vi "FPGA.vi"() -> ()   [LabVIEW 2020]
uses:
  <vilib>/Platform/TimedLoop/XDataNode/timing_clust.ctl
  <vilib>/Platform/TimedLoop/XDataNode/nitl_modes.ctl
  <vilib>/Platform/TimedLoop/XDataNode/wakeup.ctl
  <vilib>/rvi/Analysis/measure/FFT/simModelSupport/niFPGA FFT Sim Properties.ctl
  <vilib>/rvi/Analysis/measure/FFT/simModelSupport/niFPGA FFT Sim Types.ctl
  <vilib>/rvi/Analysis/measure/FFT/simModelSupport/niFpgaFFTSimArithmeticProperties.ctl
  <vilib>/rvi/Analysis/measure/FFT/simModelSupport/niFpgaFFTSimDfxp.ctl
  <vilib>/fxp/LVFixedPointQuantizationPolicyTypeDef.ctl
  <vilib>/rvi/DataTransferAndStorage/Container/Common/niFpgaContainerGetUniqueNameForEmu.vi
  <vilib>/rvi/DataTransferAndStorage/Container/Common/niFpgaContainerSetEmuInfo.vi
  <vilib>/rvi/eio/common/nirviEmuReportErrorAndStop.vi
  <vilib>/rvi/eio/common/nirviEmuTemplateMethod_errors.vi
  <vilib>/rvi/DataTransferAndStorage/Container/Common/niFpgaContainerExecOnDevCompGetState.vi
  <vilib>/rvi/Emulation/niFpgaEmulationIsFPGAContextNoSignature.vi
  <vilib>/rvi/Emulation/niFpgaSctlEmulationGetInTimedLoop.vi
  <vilib>/rvi/errors/niFpgaSetErrorForExecOnDevCompSimple.vi
  <vilib>/rvi/FIFO/Fifo_Resource/nirvififoEmulationSetSize.vi
  <vilib>/rvi/FIFO/Fifo_Resource/nirviFifoEmulationQueueMgr.vi
  <instcachedir>/0/nirviFifoEmulationQueueMgr_E5CAEC123FF24DC58D834DCA3CDAA9B5.lvgen/nirviFifoEmulationQueueMgr_E5CAEC123FF24DC58D834DCA3CDAA9B5_003.vi
  <vilib>/rvi/FIFO/Fifo_Resource/nirvififoEmulationDetermineInputValidOut.vi
  <vilib>/rvi/FIFO/Fifo_Resource/nirvififoEmulationCreateLock.vi
  <vilib>/rvi/Emulation/niFpgaProcessEmulError.vi
  <vilib>/rvi/FIFO/Fifo_Resource/nirvififoEmulationObtainLock.vi
  <vilib>/rvi/FIFO/Fifo_Resource/nirvififoEmulationReleaseLock.vi
  <vilib>/rvi/occurrence/nirviWaitOnOccurrenceBase.vi
  <vilib>/rvi/errors/nirviReportUnexpectedCaseInternalError.vi
  <vilib>/rvi/errors/nirviReportUnexpectedCaseInternalError (U32).vi
  <vilib>/Utility/error.llb/Clear Errors.vi
  <vilib>/rvi/interface/RandomDataEmulation/niFpgaRandomDataHandleErrors.vi
  <vilib>/rvi/Emulation/niFpgaEmulationReportErrorSimple.vi
  <vilib>/rvi/Emulation/niFpgaGetClockAttributes.vi
  <vilib>/rvi/Emulation/niFpgaCriticalErrorInLSC.vi
  <vilib>/rvi/Analysis/measure/FFT/simModelSupport/niFpgaFFTSimModelCore.vi
  <vilib>/rvi/LocalResourceManager/LocalResourceManager.xnode
  <vilib>/eio/EIONode/EIONode.xnode
  <vilib>/rvi/DataTransferAndStorage/Container/XNode/niFpgaContainer.xnode
  <vilib>/rvi/FIFO/Fifo_Resource/niFpgaFifoEmulationRefIn.vi
  <vilib>/Platform/TimedLoop/XDataNode/XDataNode.xnode
  <vilib>/rvi/interface/RandomDataEmulation/nirviRandomDataFpgaReadWriteTemplate.vi
  <vilib>/rvi/Analysis/measure/FFT/XNode/niFpgaFFT.xnode
  <vilib>/rvi/FXPMathLib/FxpInterpret/XNode/nifxpmath_Interpret.xnode
  <vilib>/Platform/TimedLoop/XDataNode/XDNodeRunTimeDep.lvlib
panel:
  out "Timed Out? FIFO out index 2":bool
  out "Timed Out? FIFO out IMG 2":bool
  out "Timed Out? FIFO out REAL 2":bool
  in  "FFT loop iterations":i32
  in  "auto stop":bool
  out "FFT time (uSec)":u32
  out "data collection time (uSec)":u32
  in  "Loop number":i32
  out "Element":fxp<+/-,24,7>
  in  "Rate (uSec)":u32 caption="Count(uSec)"
  out "Timed Out?":bool
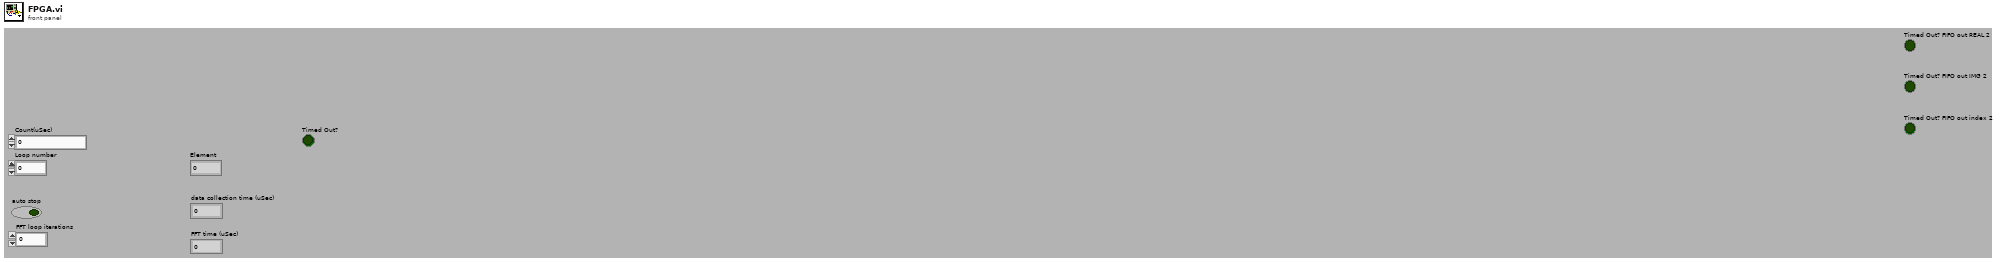
[diagram p1: front panel]
types:
  T1 = typedef "XDNodeRunTimeDep.lvlib/timing_clust.ctl" = cluster{"Expected End [f-1]":u64, "Actual End [f-1]":u64, "Finished Late? [f-1]":bool, "Expected End [i-1]":u64, "Actual End [i-1]":u64, "Finished Late? [i-1]":bool, "Expected Start [i]":u64, "Actual Start [i]":u64, "Expected Start [f]":u64, "Actual Start [f]":u64, "Source Name":string, "Structure Name":string, "Period":i64, "Deadline":i64, "Offset":i64, "Start":i64, "Priority":i32, "Timeout":i32, "Mode":T2, "Wakeup Reason":T3, "Error":errorcluster, "Source Type":string, "Secondary Source Type":string, "Global End Time":u64, "Global Start Time":u64, "Frame Duration":u64, "Iteration Duration":u64, "Assigned CPU":i32, "I/O Scan Engine Mode":u32}
  T2 = typedef "XDNodeRunTimeDep.lvlib/nitl_modes.ctl" = enum32{"No Change", "Process missed periods, maintain original phase", "Discard missed periods, maintain original phase", "Process missed periods, ignore original phase", "Discard missed periods, ignore original phase"}
  T3 = typedef "XDNodeRunTimeDep.lvlib/wakeup.ctl" = enum32{"Normal", "Aborted", "Asynchronous wakeup", "Timing source error", "Timed loop error", "Timeout"}
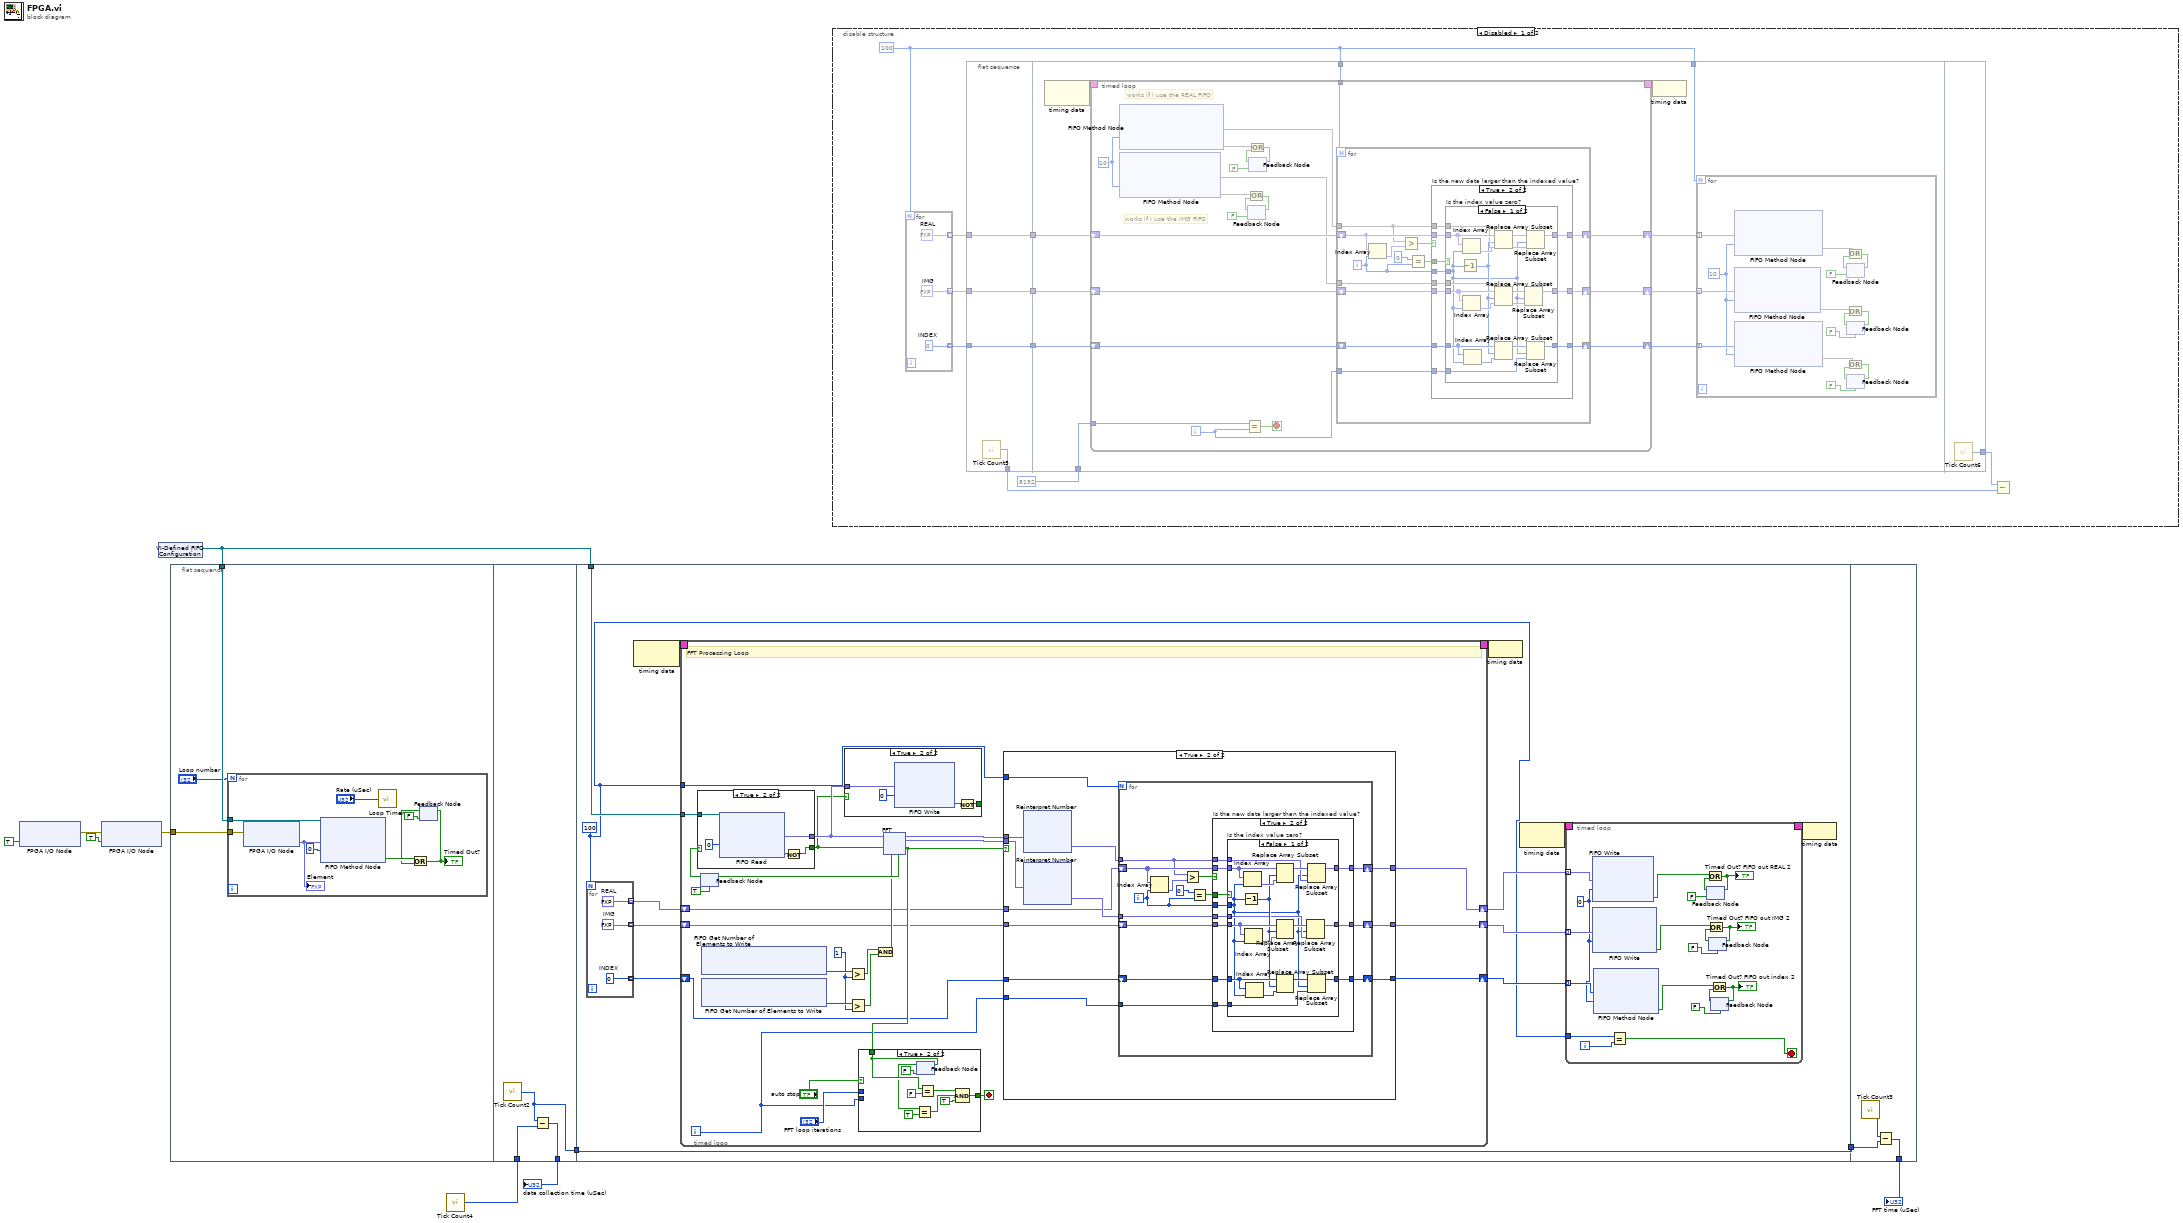
[diagram p0: block diagram]
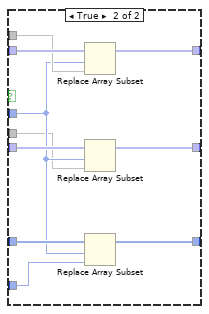
[diagram p3: hidden frame]
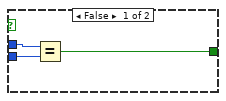
[diagram p5: hidden frame]
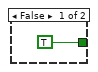
[diagram p6: hidden frame]
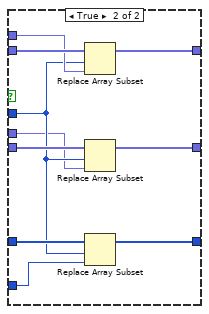
[diagram p9: hidden frame]
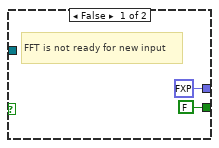
[diagram p10: hidden frame]
diagram:
  n1 = xnode "FPGA I/O Node"("Mod1/Stop"=TRUE) -> ("error out"=w3:errorcluster)  [unwired: 2 in, 1 out]
  n2 = xnode "FPGA I/O Node"("error in"=w3, "Mod1/Start"=TRUE) -> ("error out"=w2:errorcluster)  [unwired: 1 in, 1 out]
  n3 = xnode "VI-Defined FIFO Configuration"() -> ("FIFO Out"=w10:refnum<k21>)
  n4 = flat-sequence {
    tunnel: w10 -> [w13]
    tunnel: w2 -> [w11]
    tunnel: [w25] -> w9
    tunnel: [w24] -> w8
    tunnel: w1 -> [w23]
    tunnel: w10 -> [w36]
    tunnel: w8 -> [w35]
    tunnel: [w35] -> w7
    tunnel: w7 -> [w216]
    tunnel: [w215] -> w6
    frame #0 {
      n5 = for {
        N: "Loop number" -> [_]
        tunnel: w13 -> [w22]
        tunnel: w11 -> [w21]
        n6 = xnode "FPGA I/O Node"("error in"=w21) -> ("Mod1/AI0"=w15:fxp<+/-,24,7>)  [unwired: 1 in, 2 out]
        "Element" <- w15
        n7 = xnode ("FIFO Method Node")("Element"=w15, "Timeout"=0, "FIFO In"=w22) -> ("Timed Out?"=w19:bool)  [unwired: 1 in, 2 out]
        n8 = call "Loop Timer"("Count(uSec)"="Rate (uSec)") -> ()  [unwired: 1 out]
        n9 = feedback #1(FALSE) -> (w18:bool)
        n10 = Or(x=w19, y=w18) -> (x .or. y?=w17:bool)
        "Timed Out?" <- w17
        n11 = feedback-in #1(w17) -> ()
      }
    }
    frame #1 {
      n12 = call "Tick Count2"() -> ("Tick Count(uSec)"=w24:u32)
      n13 = Subtract(x=w24, y=w23) -> (x-y=w25:u32)
    }
    frame #2 {
      w26 = 100
      n14 = for {
        N: w26 -> [_]
        tunnel: [w64] -> w34 mode=indexing
        tunnel: [w63] -> w29 mode=indexing
        tunnel: [w62] -> w33 mode=indexing
        w62 = fxp<+/-,32,21> 0.0  # IMG
        w63 = 0  # INDEX
        w64 = fxp<+/-,32,21> 0.0  # REAL
      }
      n15 = node-c288() -> (w38:T1)  [unwired: 1 in]
      n16 = timed-loop {
        timing: w38 -> [_]
        timing-out: [_] -> w37
        tunnel: w36 -> [w87]
        tunnel: w26 -> [w66]
        shift-right: [w67] -> w30
        shift-left: w29 -> [w65]
        shift-right: [w68] -> w32
        shift-left: w33 -> [w71]
        shift-right: [w69] -> w31
        shift-left: w34 -> [w72]
        i -> [w70]
        stop <- w77 stop-if-true
        w82 = u32 1 ("y")
        # "FFT Processing Loop"
        n17 = feedback #2(TRUE ("ready for input")) -> (w90:bool)
        n18 = case shown="True" w90 {
          tunnel: [FALSE w209] -> w79
          tunnel: [fxp<+/-,16,5> 0.0 ("Element") w210] -> w89
          tunnel: w87 -> [_ w206]
          frame False {
            # "FFT is not ready for new input"
          }
          frame True {
            n19 = xnode ("FIFO Read")("Timeout"=0, "FIFO In"=w206) -> ("Element"=w210:fxp<+/-,24,7>, "Timed Out?"=w208:bool)  [unwired: 1 out]
            n20 = Not(x=w208) -> (.not. x?=w209:bool)
          }
        }
        n21 = xnode ("FIFO Get Number of Elements to Write")() -> ("Number of Elements to Write"=w84:u32)  [unwired: 1 in, 1 out]
        n22 = xnode ("FIFO Get Number of Elements to Write")() -> ("Number of Elements to Write"=w83:u32)  [unwired: 1 in, 1 out]
        n23 = case shown="True" w79 {
          tunnel: w89 -> [_ w104]
          tunnel: [TRUE ("Timed Out?") w105] -> _
          frame False {
          }
          frame True {
            n24 = xnode ("FIFO Write")("Element"=w104, "Timeout"=0) -> ("Timed Out?"=w106:bool)  [unwired: 1 in, 1 out]
            n25 = Not(x=w106) -> (.not. x?=w105:bool)
          }
        }
        n26 = Greater?(x=w84, y=w82) -> (0:w81:bool)
        n27 = Greater?(x=w83, y=w82) -> (0:w80:bool)
        n28 = Compound Arithmetic op=AND(w81, w80) -> (w78:bool)
        n29 = xnode "FFT"("real data in"=w89, "input valid"=w79, "ready for output"=w78) -> ("ready for input"=w88:bool, "real data out"=w86:fxp<+/-,32,21>, "imaginary data out"=w76:fxp<+/-,32,21>, "output valid"=w73:bool)  [unwired: 2 in, 1 out]
        n30 = feedback-in #2(w88) -> ()
        n31 = case shown="True" "auto stop" {
          tunnel: w73 -> [_ w101]
          tunnel: [w91 w94] -> w77
          tunnel: w70 -> [w93 _]
          tunnel: "FFT loop iterations" -> [w92 _]
          frame False {
            n32 = Equal?(x=w92, y=w93) -> (x = y?=w91:bool)
          }
          frame True {
            n33 = feedback #3(FALSE) -> (w98:bool)
            n34 = Equal?(x=w98, y=TRUE) -> (x = y?=w96:bool)
            n35 = feedback-in #3(w101) -> ()
            n36 = Equal?(x=w101, y=FALSE) -> (x = y?=w97:bool)
            n37 = Compound Arithmetic op=AND(w97, w96, TRUE ("value")) -> (w94:bool)
          }
        }
        n38 = case shown="True" w73 {
          tunnel: w86 -> [_ w148]
          tunnel: w76 -> [_ w147]
          tunnel: w72 -> [w136 w144]
          tunnel: w71 -> [w135 w143]
          tunnel: w65 -> [w134 w142]
          tunnel: w70 -> [_ w141]
          tunnel: [w136 w140] -> w69
          tunnel: [w135 w139] -> w68
          tunnel: [w134 w138] -> w67
          tunnel: w66 -> [_ w137]
          frame False {
          }
          frame True {
            n39 = xnode "Reinterpret Number"("x"=w148) -> ("y"=w146:fxp<+/-,32,21>)
            n40 = xnode "Reinterpret Number"("x"=w147) -> ("y"=w145:fxp<+/-,32,21>)
            n41 = for {
              N: w137 -> [_]
              tunnel: w146 -> [w159]
              shift-right: [w158] -> w140
              shift-left: w144 -> [w160]
              tunnel: w141 -> [w156]
              shift-right: [w154] -> w138
              shift-left: w142 -> [w155]
              shift-right: [w151] -> w139
              shift-left: w143 -> [w150]
              tunnel: w145 -> [w149]
              i -> [w157]
              n42 = Index Array(array=w160, index=w157) -> (element=w162:fxp<+/-,32,21>)
              n43 = Greater?(x=w159, y=w162) -> (0:w161:bool)
              n44 = Equal?(x=0, y=w157) -> (x = y?=w152:bool)
              n45 = case "Is the new data larger than the indexed value?" shown="True" w161 {
                tunnel: w160 -> [w165 w175]
                tunnel: w152 -> [_ w176]
                tunnel: w159 -> [_ w174]
                tunnel: w157 -> [_ w173]
                tunnel: [w165 w172] -> w158
                tunnel: w156 -> [_ w171]
                tunnel: w155 -> [w164 w170]
                tunnel: [w164 w169] -> w154
                tunnel: [w163 w168] -> w151
                tunnel: w150 -> [w163 w167]
                tunnel: w149 -> [_ w166]
                frame False {
                }
                frame True {
                  n46 = case "Is the index value zero?" shown="False" w176 {
                    tunnel: w175 -> [w193 w203]
                    tunnel: w174 -> [w190 w202]
                    tunnel: w173 -> [w177 w196]
                    tunnel: [w189 w201] -> w172
                    tunnel: w171 -> [w184 w200]
                    tunnel: w170 -> [w186 w199]
                    tunnel: [w185 w198] -> w169
                    tunnel: [w179 w194] -> w168
                    tunnel: w167 -> [w183 w197]
                    tunnel: w166 -> [w178 w195]
                    frame False {
                      n47 = Decrement(x=w177) -> (x-1=w181:i32)
                      n48 = Index Array(array=w193, index=w177) -> (element=w192:fxp<+/-,32,21>)
                      n49 = Index Array(array=w183, index=w177) -> (element=w182:fxp<+/-,32,21>)
                      n50 = Index Array(array=w186, index=w177) -> (element=w188:i32)
                      n51 = Replace Array Subset(array=w193, new element=w192, index=w181) -> (w191:fxp<+/-,32,21>[])
                      n52 = Replace Array Subset(array=w183, new element=w182, index=w181) -> (w180:fxp<+/-,32,21>[])
                      n53 = Replace Array Subset(array=w186, new element=w188, index=w181) -> (w187:i32[])
                      n54 = Replace Array Subset(array=w180, new element=w178, index=w177) -> (w179:fxp<+/-,32,21>[])
                      n55 = Replace Array Subset(array=w191, new element=w190, index=w177) -> (w189:fxp<+/-,32,21>[])
                      n56 = Replace Array Subset(array=w187, new element=w184, index=w177) -> (w185:i32[])
                    }
                    frame True {
                      n57 = Replace Array Subset(array=w203, new element=w202, index=w196) -> (w201:fxp<+/-,32,21>[])
                      n58 = Replace Array Subset(array=w197, new element=w195, index=w196) -> (w194:fxp<+/-,32,21>[])
                      n59 = Replace Array Subset(array=w199, new element=w200, index=w196) -> (w198:i32[])
                    }
                  }
                }
              }
            }
          }
        }
      }
      n60 = node-c288(w37) -> ()
      n61 = node-c288() -> (w28:T1)  [unwired: 1 in]
      n62 = timed-loop {
        tunnel: w32 -> [w57] mode=indexing
        tunnel: w31 -> [w56] mode=indexing
        tunnel: w30 -> [w46] mode=indexing
        timing: w28 -> [_]
        timing-out: [_] -> w27
        tunnel: w26 -> [w40]
        i -> [w41]
        stop <- w39 stop-if-true
        w45 = 0 ("Timeout")
        n63 = xnode ("FIFO Write")("Element"=w56, "Timeout"=w45) -> ("Timed Out?"=w42:bool)  [unwired: 1 in, 1 out]
        n64 = xnode ("FIFO Write")("Element"=w57, "Timeout"=w45) -> ("Timed Out?"=w43:bool)  [unwired: 1 in, 1 out]
        n65 = xnode ("FIFO Method Node")("Element"=w46, "Timeout"=w45) -> ("Timed Out?"=w44:bool)  [unwired: 1 in, 1 out]
        n66 = Equal?(x=w40, y=w41) -> (x = y?=w39:bool)
        n67 = feedback #4(FALSE) -> (w53:bool)
        n68 = Or(x=w42, y=w53) -> (x .or. y?=w54:bool)
        "Timed Out? FIFO out REAL 2" <- w54
        n69 = feedback-in #4(w54) -> ()
        n70 = feedback #5(FALSE) -> (w52:bool)
        n71 = Or(x=w43, y=w52) -> (x .or. y?=w51:bool)
        "Timed Out? FIFO out IMG 2" <- w51
        n72 = feedback-in #5(w51) -> ()
        n73 = feedback #6(FALSE) -> (w49:bool)
        n74 = Or(x=w44, y=w49) -> (x .or. y?=w48:bool)
        "Timed Out? FIFO out index 2" <- w48
        n75 = feedback-in #6(w48) -> ()
      }
      n76 = node-c288(w27) -> ()
    }
    frame #3 {
      n77 = call "Tick Count3"() -> ("Tick Count(uSec)"=w217:u32)
      n78 = Subtract(x=w217, y=w216) -> (x-y=w215:u32)
    }
  }
  n79 = call "Tick Count4"() -> ("Tick Count(uSec)"=w1:u32)
  n80 = disable-structure shown="Disabled" {
    frame Disabled {
      w219 = 100
      n81 = for {
        N: w219 -> [_]
        tunnel: [w230] -> w221 mode=indexing
        tunnel: [w229] -> w222 mode=indexing
        tunnel: [w228] -> w218 mode=indexing
        w228 = fxp<+/-,32,21> 0.0  # IMG
        w229 = 0  # INDEX
        w230 = fxp<+/-,32,21> 0.0  # REAL
      }
      n82 = flat-sequence {
        tunnel: [w234] -> w223
        tunnel: [w233] -> w227
        tunnel: w222 -> [w233]
        tunnel: [w232] -> w226
        tunnel: w221 -> [w232]
        tunnel: [w231] -> w225
        tunnel: w218 -> [w231]
        tunnel: w227 -> [w245]
        tunnel: w226 -> [w244]
        tunnel: 8192 ("samples") -> [w242]
        tunnel: w219 -> [w243]
        tunnel: w219 -> [w239]
        tunnel: w225 -> [w235]
        tunnel: [w342] -> w224
        frame #0 {
          n83 = call "Tick Count5"() -> ("Tick Count(uSec)"=w234:u32)
        }
        frame #1 {
          n84 = node-c288() -> (w241:T1)  [unwired: 1 in]
          n85 = timed-loop {
            shift-right: [w281] -> w237
            shift-left: w244 -> [w282]
            shift-right: [w280] -> w238
            shift-left: w245 -> [w279]
            tunnel: w243 -> [w278]
            tunnel: w242 -> [w276]
            timing: w241 -> [_]
            timing-out: [_] -> w240
            shift-right: [w274] -> w236
            shift-left: w235 -> [w273]
            i -> [w277]
            stop <- w275 stop-if-true
            w272 = 10 ("Timeout")
            # "works if I use the REAL FIFO"
            # "works if I use the IMG FIFO"
            n86 = xnode ("FIFO Method Node")("Timeout"=w272) -> ("Element"=w270, "Timed Out?"=w262)  [unwired: 1 in, 1 out]
            n87 = xnode ("FIFO Method Node")("Timeout"=w272) -> ("Element"=w271, "Timed Out?"=w266)  [unwired: 1 in, 1 out]
            n88 = Equal?(x=w276, y=w277) -> (x = y?=w275:bool)
            n89 = feedback #7(FALSE) -> (w267:bool)
            n90 = Or(x=w266, y=w267) -> (x .or. y?=w268:bool)
            n91 = feedback-in #7(w268) -> ()
            n92 = feedback #8(FALSE) -> (w263:bool)
            n93 = Or(x=w262, y=w263) -> (x .or. y?=w264:bool)
            n94 = feedback-in #8(w264) -> ()
            n95 = for {
              N: w278 -> [_]
              tunnel: w270 -> [w293]
              shift-right: [w292] -> w281
              shift-left: w282 -> [w294]
              tunnel: w277 -> [w290]
              shift-right: [w288] -> w280
              shift-left: w279 -> [w289]
              shift-right: [w285] -> w274
              shift-left: w273 -> [w284]
              tunnel: w271 -> [w283]
              i -> [w291]
              n96 = Index Array(array=w294, index=w291) -> (element=w296:fxp<+/-,32,21>)
              n97 = Greater?(x=w293, y=w296) -> (0:w295:bool)
              n98 = Equal?(x=0, y=w291) -> (x = y?=w286:bool)
              n99 = case "Is the new data larger than the indexed value?" shown="True" w295 {
                tunnel: w294 -> [w299 w309]
                tunnel: w286 -> [_ w310]
                tunnel: w293 -> [_ w308]
                tunnel: w291 -> [_ w307]
                tunnel: [w299 w306] -> w292
                tunnel: w290 -> [_ w305]
                tunnel: w289 -> [w298 w304]
                tunnel: [w298 w303] -> w288
                tunnel: [w297 w302] -> w285
                tunnel: w284 -> [w297 w301]
                tunnel: w283 -> [_ w300]
                frame False {
                }
                frame True {
                  n100 = case "Is the index value zero?" shown="False" w310 {
                    tunnel: w309 -> [w327 w337]
                    tunnel: w308 -> [w324 w336]
                    tunnel: w307 -> [w311 w330]
                    tunnel: [w323 w335] -> w306
                    tunnel: w305 -> [w318 w334]
                    tunnel: w304 -> [w320 w333]
                    tunnel: [w319 w332] -> w303
                    tunnel: [w313 w328] -> w302
                    tunnel: w301 -> [w317 w331]
                    tunnel: w300 -> [w312 w329]
                    frame False {
                      n101 = Decrement(x=w311) -> (x-1=w315:i32)
                      n102 = Index Array(array=w327, index=w311) -> (element=w326:fxp<+/-,32,21>)
                      n103 = Index Array(array=w317, index=w311) -> (element=w316:fxp<+/-,32,21>)
                      n104 = Index Array(array=w320, index=w311) -> (element=w322:i32)
                      n105 = Replace Array Subset(array=w327, new element=w326, index=w315) -> (w325:fxp<+/-,32,21>[])
                      n106 = Replace Array Subset(array=w317, new element=w316, index=w315) -> (w314:fxp<+/-,32,21>[])
                      n107 = Replace Array Subset(array=w320, new element=w322, index=w315) -> (w321:i32[])
                      n108 = Replace Array Subset(array=w314, new element=w312, index=w311) -> (w313:fxp<+/-,32,21>[])
                      n109 = Replace Array Subset(array=w325, new element=w324, index=w311) -> (w323:fxp<+/-,32,21>[])
                      n110 = Replace Array Subset(array=w321, new element=w318, index=w311) -> (w319:i32[])
                    }
                    frame True {
                      n111 = Replace Array Subset(array=w337, new element=w336, index=w330) -> (w335:fxp<+/-,32,21>[])
                      n112 = Replace Array Subset(array=w331, new element=w329, index=w330) -> (w328:fxp<+/-,32,21>[])
                      n113 = Replace Array Subset(array=w333, new element=w334, index=w330) -> (w332:i32[])
                    }
                  }
                }
              }
            }
          }
          n114 = node-c288(w240) -> ()
          n115 = for {
            N: w239 -> [_]
            tunnel: w238 -> [w261] mode=indexing
            tunnel: w237 -> [w260] mode=indexing
            tunnel: w236 -> [w259] mode=indexing
            w258 = 10 ("Timeout")
            n116 = xnode ("FIFO Method Node")("Element"=w261, "Timeout"=w258) -> ("Timed Out?"=w246)  [unwired: 1 in, 1 out]
            n117 = xnode ("FIFO Method Node")("Element"=w260, "Timeout"=w258) -> ("Timed Out?"=w254)  [unwired: 1 in, 1 out]
            n118 = xnode ("FIFO Method Node")("Element"=w259, "Timeout"=w258) -> ("Timed Out?"=w250)  [unwired: 1 in, 1 out]
            n119 = feedback #9(FALSE) -> (w255:bool)
            n120 = Or(x=w254, y=w255) -> (x .or. y?=w256:bool)
            n121 = feedback-in #9(w256) -> ()
            n122 = feedback #10(FALSE) -> (w253:bool)
            n123 = Or(x=w250, y=w253) -> (x .or. y?=w252:bool)
            n124 = feedback-in #10(w252) -> ()
            n125 = feedback #11(FALSE) -> (w249:bool)
            n126 = Or(x=w246, y=w249) -> (x .or. y?=w248:bool)
            n127 = feedback-in #11(w248) -> ()
          }
        }
        frame #2 {
          n128 = call "Tick Count6"() -> ("Tick Count(uSec)"=w342:u32)
        }
      }
      n129 = Subtract(x=w224, y=w223) -> ()  [unwired: 1 out]
    }
    frame Enabled {
    }
  }
  "data collection time (uSec)" <- w9
  "FFT time (uSec)" <- w6
